vi "_builtins_icon.vi"(8 "error in (no error)":errorcluster, 10 "Args":string[](array[string]), 11 "VI Refnum in":refnum<vi>) -> (0 "error out":errorcluster, 3 "VI Refnum out":refnum<vi>)   [LabVIEW 2019, in "Script.lvlib"]
doc: "Updates the VI Icon formatted as.\n\n--icon [TEXT1 TEXT2 TEXT3 TEXT4] [options]\n\noptions:\n -bc BORDER_COLOR=black\n -c FILL_COLOR=none\n -g GLYPH=[none|get|set|create|config|read|write|cmd|tlm|destroy|ctl|ctl_cmd|ctl_tlm]\n -h HEADER=[owner|TEXT]\n -hc HEADER_FILL_COLOR=none\n -hj HEADER_JUSTIFY=[center|left|right]\n -htc HEADER_TEXT_COLOR=black\n -tc TEXT_COLOR=black\n -tj TEXT_JUSTIFY=[center|left|right]\n\nExample: \"--icon TEMP DATA -h DRIVER -hc ? -g read\"\n\nColors can be a X11 color names (\"cyan\"), html color code (\"#ffdd23\") or random (\"?\")\n\nCreated by: Ryan Pacini"
uses:
  Script.lvlib
  _builtins_icon.ctl
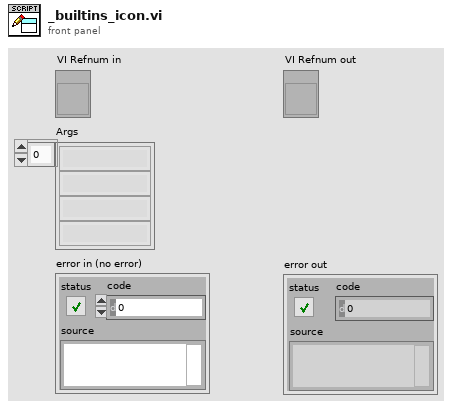
[diagram p1: front panel]
types:
  T1 = cluster{"text":string, "fg":u32, "bg":u32, "justify":enum8{"center", "left", "right"}, "owner":bool}
  T2 = cluster{"text":string[], "fg":u32, "justify":enum8{"center", "left", "right"}}
  T3 = enum8{"none", "get", "set", "create", "config", "read", "write", "cmd", "tlm", "destroy", "ctl", "ctl_cmd", "ctl_tlm"}
  T4 = typedef "Script.lvlib/_builtins_icon.ctl" = cluster{"fg":u32, "bg":u32, "glyph":enum8{"none", "get", "set", "create", "config", "read", "write", "cmd", "tlm", "destroy", "ctl", "ctl_cmd", "ctl_tlm"}, "header":cluster{"text":string, "fg":u32, "bg":u32, "justify":enum8{"center", "left", "right"}, "owner":bool}, "text":cluster{"text":string[], "fg":u32, "justify":enum8{"center", "left", "right"}}}
  T5 = typedef "imagedata.ctl" = cluster{"image type":i32, "image depth":i32, "image":u8[], "mask":u8[], "colors":u32[], "Rectangle":cluster{"left":i16, "top":i16, "right":i16, "bottom":i16}}
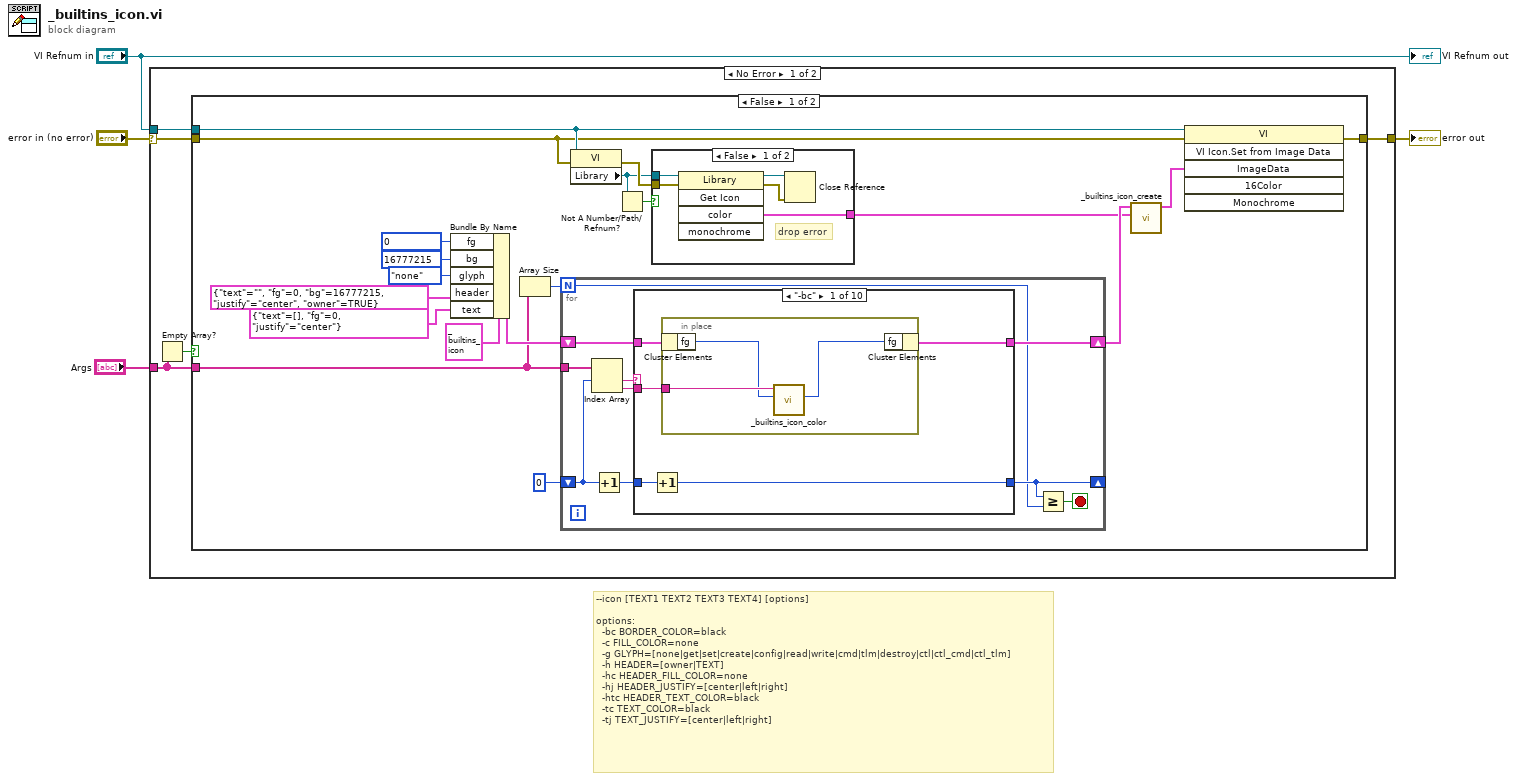
[diagram p0: block diagram]
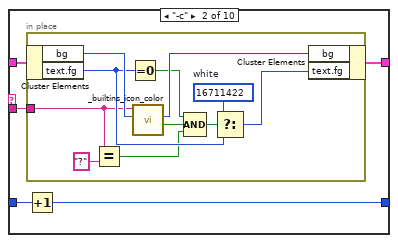
[diagram p3: hidden frame]
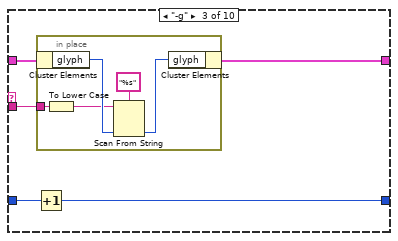
[diagram p4: hidden frame]
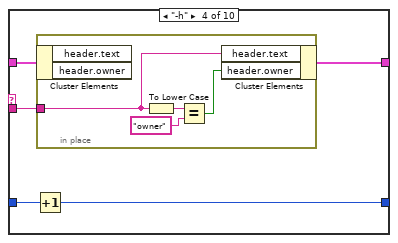
[diagram p5: hidden frame]
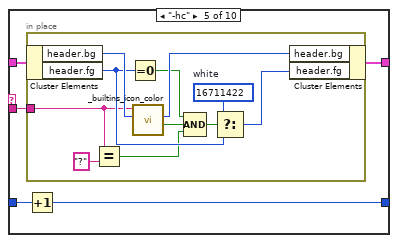
[diagram p6: hidden frame]
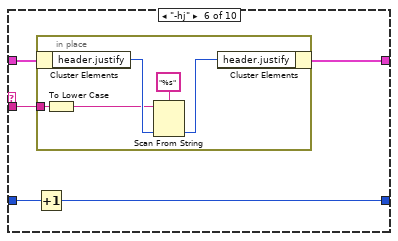
[diagram p7: hidden frame]
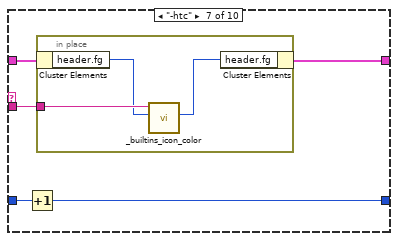
[diagram p8: hidden frame]
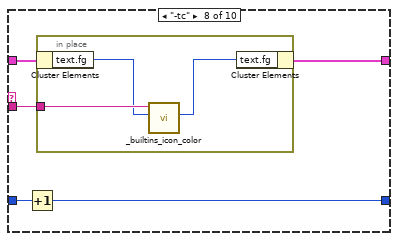
[diagram p9: hidden frame]
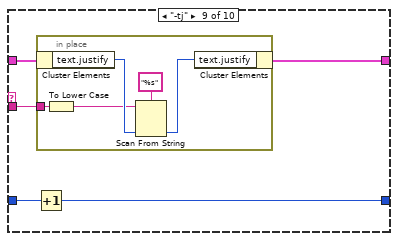
[diagram p10: hidden frame]
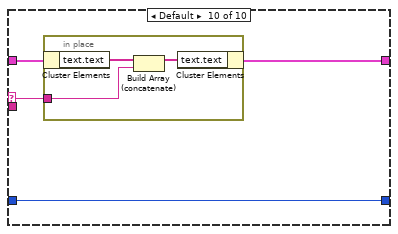
[diagram p11: hidden frame]
diagram:
  # "--icon [TEXT1 TEXT2 TEXT3 TEXT4] [options]\n\noptions:\n  -bc BORDER_COLOR=black\n  -c FILL_COLOR=none\n  -g GLYPH=[none|get|set|create|config|read|write|cmd|tlm|destroy|ctl|ctl_cmd|ctl_tlm]\n  -h HEADER=[owner|TEXT]\n  -hc HEADER_FILL_COLOR=none\n  -hj HEADER_JUSTIFY=[center|left|right]\n  -htc HEADER_TEXT_COLOR=black\n  -tc TEXT_COLOR=black\n  -tj TEXT_JUSTIFY=[center|left|right]"
  n1 = case shown="No Error" "error in (no error)" {
    selector: "error in (no error)" -> [w7 w147]
    tunnel: "VI Refnum in" -> [w8 _]
    tunnel: [w9 w147] -> w1
    tunnel: "Args" -> [w6 _]
    frame No Error {
      n2 = Empty Array?(array=w6) -> (empty?=w5:bool)
      n3 = case shown="False" w5 {
        tunnel: [w28 w146] -> w9
        tunnel: w8 -> [w25 _]
        tunnel: w6 -> [w16 _]
        tunnel: w7 -> [w14 w146]
        frame False {
          n4 = Bundle By Name(cluster=T4 {"fg"=0, "bg"=16777215, "glyph"=enum."none", "header"={"text"="", "fg"=0, "bg"=16777215, "justify"=enum."center", "owner"=FALSE}, "text"={"text"=[], "fg"=0, "justify"=enum."center"}} ("icon"), "fg"=u32 0, "bg"=u32 16777215, "glyph"=T3."none", "header"=T1 {"text"="", "fg"=0, "bg"=16777215, "justify"=enum."center", "owner"=TRUE}, "text"=T2 {"text"=[], "fg"=0, "justify"=enum."center"}) -> (w23:T4)
          n5 = Array Size(array=w16) -> (size(s)=w15:i32)
          n6 = for {
            N: w15 -> [w34]
            shift-right: [w43] -> w18
            shift-left: w23 -> [w42]
            shift-right: [w36] -> _
            shift-left: 0 -> [w39]
            tunnel: w16 -> [w41]
            stop <- w35 stop-if-true
            n7 = Index Array(array=w41, index #1=w39) -> (element #1=w40:string, element #2=w38:string)  [unwired: 1 in]
            n8 = Increment(x=w39) -> (x+1=w37:i32)
            n9 = case shown="\"-bc\"" w40 {
              selector: w40 -> [_ _ _ _ _ _ _ _ _ w141]
              tunnel: [w45 w53 w69 w79 w88 w104 w114 w122 w130 w140] -> w43
              tunnel: w42 -> [w46 w54 w70 w80 w89 w105 w115 w123 w131 w142]
              tunnel: [w44 w52 w68 w78 w87 w103 w113 w121 w129 w139] -> w36
              tunnel: w37 -> [w48 w56 w72 w82 w91 w107 w117 w125 w133 w139]
              tunnel: w38 -> [w47 w55 w71 w81 w90 w106 w116 w124 w132 _]
              frame "-bc" {
                n10 = Increment(x=w48) -> (x+1=w44:i32)
                n11 = in-place {
                  in-place-border: w47 -> [w51]
                  n12 = in-place-cluster #1(w46) -> ("fg"=w50:u32)
                  n13 = call "_builtins_icon_color.vi"("Default Color (none)"=w50, "color (name, #ddeeff, ?)"=w51) -> ("Color"=w49:u32)  [unwired: 7 in, 2 out]
                  n14 = in-place-cluster #1("fg"=w49) -> (w45:T4)
                }
              }
              frame "-c" {
                n15 = in-place {
                  in-place-border: w55 -> [w59]
                  w61 = u32 16711422  # white
                  n16 = in-place-cluster #2(w54) -> ("bg"=w67:u32, "text.fg"=w62:u32)
                  n17 = Equal?(x=w59, y="?") -> (x = y?=w57:bool)
                  n18 = Equal To 0?(x=w62) -> (x = 0?=w64:bool)
                  n19 = call "_builtins_icon_color.vi"("Default Color (none)"=w67, "color (name, #ddeeff, ?)"=w59) -> ("Invert Text?"=w65:bool, "Color"=w66:u32)  [unwired: 7 in, 1 out]
                  n20 = Compound Arithmetic op=AND(w64, w65, w57) -> (w63:bool)
                  n21 = Select(t=w61, s=w63, f=w62) -> (s? t:f=w60:u32)
                  n22 = in-place-cluster #2("bg"=w66, "text.fg"=w60) -> (w53:T4)
                }
                n23 = Increment(x=w56) -> (x+1=w52:i32)
              }
              frame "-g" {
                n24 = Increment(x=w72) -> (x+1=w68:i32)
                n25 = in-place {
                  in-place-border: w71 -> [w76]
                  n26 = in-place-cluster #3(w70) -> ("glyph"=w77:T3)
                  n27 = To Lower Case(string=w76) -> (all lower case string=w74:string)
                  n28 = Scan From String(format string="%s", input string=w74, default 1=w77) -> (output 1=w73:T3)  [unwired: 2 in, 3 out]
                  n29 = in-place-cluster #3("glyph"=w73) -> (w69:T4)
                }
              }
              frame "-h" {
                n30 = Increment(x=w82) -> (x+1=w78:i32)
                n31 = in-place {
                  in-place-border: w81 -> [w86]
                  n32 = in-place-cluster #4(w80) -> ()  [unwired: 2 out]
                  n33 = To Lower Case(string=w86) -> (all lower case string=w85:string)
                  n34 = Equal?(x=w85, y="owner") -> (x = y?=w83:bool)
                  n35 = in-place-cluster #4("header.text"=w86, "header.owner"=w83) -> (w79:T4)
                }
              }
              frame "-hc" {
                n36 = in-place {
                  in-place-border: w90 -> [w94]
                  w96 = u32 16711422  # white
                  n37 = in-place-cluster #5(w89) -> ("header.bg"=w102:u32, "header.fg"=w97:u32)
                  n38 = Equal?(x=w94, y="?") -> (x = y?=w92:bool)
                  n39 = Equal To 0?(x=w97) -> (x = 0?=w99:bool)
                  n40 = call "_builtins_icon_color.vi"("Default Color (none)"=w102, "color (name, #ddeeff, ?)"=w94) -> ("Invert Text?"=w100:bool, "Color"=w101:u32)  [unwired: 7 in, 1 out]
                  n41 = Compound Arithmetic op=AND(w99, w100, w92) -> (w98:bool)
                  n42 = Select(t=w96, s=w98, f=w97) -> (s? t:f=w95:u32)
                  n43 = in-place-cluster #5("header.bg"=w101, "header.fg"=w95) -> (w88:T4)
                }
                n44 = Increment(x=w91) -> (x+1=w87:i32)
              }
              frame "-hj" {
                n45 = Increment(x=w107) -> (x+1=w103:i32)
                n46 = in-place {
                  in-place-border: w106 -> [w111]
                  n47 = in-place-cluster #6(w105) -> ("header.justify"=w112:enum8{"center", "left", "right"})
                  n48 = To Lower Case(string=w111) -> (all lower case string=w109:string)
                  n49 = Scan From String(format string="%s", input string=w109, default 1=w112) -> (output 1=w108:enum8{"center", "left", "right"})  [unwired: 2 in, 3 out]
                  n50 = in-place-cluster #6("header.justify"=w108) -> (w104:T4)
                }
              }
              frame "-htc" {
                n51 = Increment(x=w117) -> (x+1=w113:i32)
                n52 = in-place {
                  in-place-border: w116 -> [w120]
                  n53 = in-place-cluster #7(w115) -> ("header.fg"=w119:u32)
                  n54 = call "_builtins_icon_color.vi"("Default Color (none)"=w119, "color (name, #ddeeff, ?)"=w120) -> ("Color"=w118:u32)  [unwired: 7 in, 2 out]
                  n55 = in-place-cluster #7("header.fg"=w118) -> (w114:T4)
                }
              }
              frame "-tc" {
                n56 = Increment(x=w125) -> (x+1=w121:i32)
                n57 = in-place {
                  in-place-border: w124 -> [w128]
                  n58 = in-place-cluster #8(w123) -> ("text.fg"=w127:u32)
                  n59 = call "_builtins_icon_color.vi"("Default Color (none)"=w127, "color (name, #ddeeff, ?)"=w128) -> ("Color"=w126:u32)  [unwired: 7 in, 2 out]
                  n60 = in-place-cluster #8("text.fg"=w126) -> (w122:T4)
                }
              }
              frame "-tj" {
                n61 = Increment(x=w133) -> (x+1=w129:i32)
                n62 = in-place {
                  in-place-border: w132 -> [w137]
                  n63 = in-place-cluster #9(w131) -> ("text.justify"=w138:enum8{"center", "left", "right"})
                  n64 = To Lower Case(string=w137) -> (all lower case string=w135:string)
                  n65 = Scan From String(format string="%s", input string=w135, default 1=w138) -> (output 1=w134:enum8{"center", "left", "right"})  [unwired: 2 in, 3 out]
                  n66 = in-place-cluster #9("text.justify"=w134) -> (w130:T4)
                }
              }
              frame Default {
                n67 = in-place {
                  in-place-border: w141 -> [w144]
                  n68 = in-place-cluster #10(w142) -> ("text.text"=w145:string[])
                  n69 = Build Array (concatenate)(w145, w144) -> (w143:string[])
                  n70 = in-place-cluster #10("text.text"=w143) -> (w140:T4)
                }
              }
            }
            n71 = Greater Or Equal?(x=w36, y=w34) -> (x >= y?=w35:bool)
          }
          n72 = property class="VI"(reference=w25, error in=w14) -> (error out=w26:errorcluster, "Library"=w11:refnum<vi>)  [unwired: 1 out]
          n73 = Not A Number/Path/Refnum?(number/path/refnum=w11) -> (NaN/Path/Refnum?=w10:bool)
          n74 = case shown="False" w10 {
            tunnel: w11 -> [w33 _]
            tunnel: w26 -> [w32 _]
            tunnel: [w29 _] -> w12
            frame False {
              # "drop error"
              n75 = invoke class="Library" method="Get Icon"(reference=w33, error in=w32) -> (reference out=w31:refnum<vi>, error out=w30:errorcluster, "color"=w29:T5)  [unwired: 3 in, 2 out]
              n76 = Close Reference(reference=w31, error in (no error)=w30) -> ()  [unwired: 1 out]
            }
            frame True {
            }
          }
          n77 = call "_builtins_icon_create.vi"("owner image"=w12, "icon"=w18) -> ("Image Data"=w27:T5)  [unwired: 9 in]
          n78 = invoke class="VI" method="VI Icon.Set from Image Data"(reference=w25, error in=w14, "ImageData"=w27) -> (error out=w28:errorcluster)  [unwired: 3 in, 5 out]
        }
        frame True {
        }
      }
    }
    frame Error {
    }
  }
  "error out" <- w1
  "VI Refnum out" <- "VI Refnum in"
